vi "parseCommand.vi"(8 "error in (no error)":errorcluster, 10 "CMDString":string, 11 "CommandParser in":refnum<class "CommandParser.lvclass">) -> (0 "error out":errorcluster, 1 "parameter":variant, 2 "MonoCommand":T1, 3 "CommandParser out":refnum<class "CommandParser.lvclass">)   [LabVIEW 2016, in "CommandParser.lvclass"]
uses:
  CommandParser.lvclass
  Typedefs/MonoCommand.ctl
  Typedefs/wavelength.ctl
  Typedefs/slitPosition.ctl
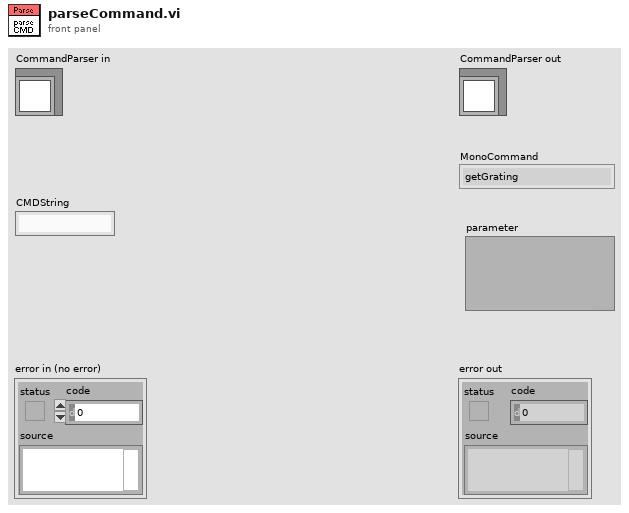
[diagram p1: front panel]
types:
  T1 = typedef "MonoCommand.ctl" = enum16{"getGrating", "getFrontEntranceSlitPosition", "getFrontExitSlitPosition", "getWavelength", "setWavelength", "setGrating", "setFrontEntranceSlitPosition", "setFrontExitSlitPosition", "calibrateWavelength", "Unknown"}
  T2 = typedef "wavelength.ctl" = dbl
  T3 = typedef "slitPosition.ctl" = dbl
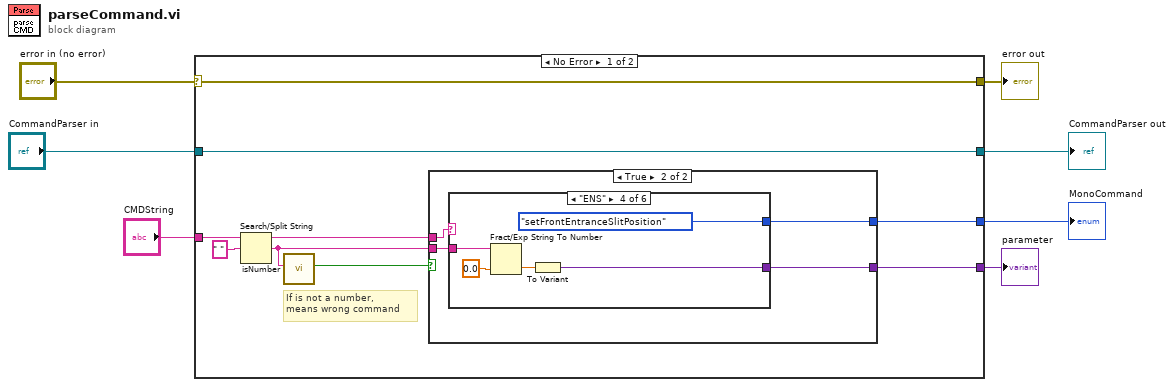
[diagram p0: block diagram]
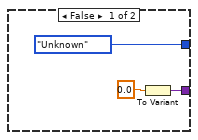
[diagram p2: hidden frame]
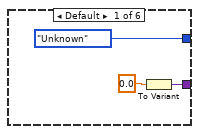
[diagram p3: hidden frame]
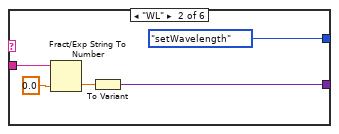
[diagram p4: hidden frame]
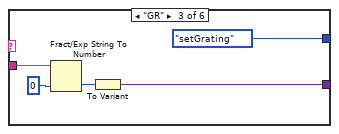
[diagram p5: hidden frame]
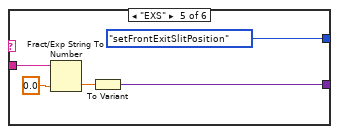
[diagram p6: hidden frame]
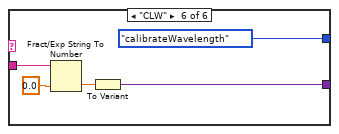
[diagram p7: hidden frame]
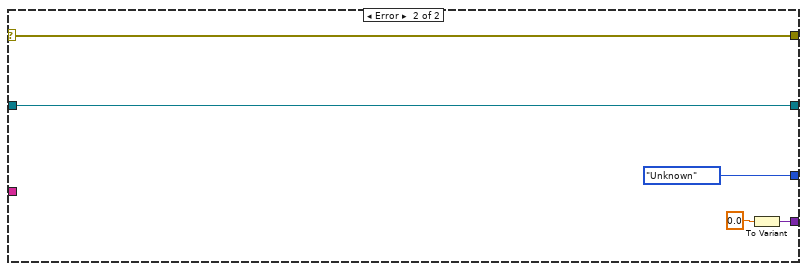
[diagram p8: hidden frame]
diagram:
  n1 = case shown="No Error" "error in (no error)" {
    selector: "error in (no error)" -> [w15 w56]
    tunnel: [w15 w56] -> w6
    tunnel: [w16 w55] -> w4
    tunnel: "CommandParser in" -> [w16 w55]
    tunnel: "CMDString" -> [w13 _]
    tunnel: [w14 MonoCommand."Unknown" ("MonoCommand")] -> w2
    tunnel: [w10 w52] -> w1
    frame No Error {
      # "If is not a number, \nmeans wrong command"
      n2 = Search/Split String(string=w13, search string/char (-)=" ") -> (substring before match=w11:string, match + rest of string=w8:string)  [unwired: 1 in, 1 out]
      n3 = call "isNumber.vi"("string"=w8) -> ("isNumber?"=w9:bool)  [unwired: 8 in, 2 out]
      n4 = case shown="True" w9 {
        tunnel: [MonoCommand."Unknown" ("MonoCommand") w23] -> w14
        tunnel: w11 -> [_ w22]
        tunnel: [w18 w21] -> w10
        tunnel: w8 -> [_ w20]
        frame False {
          n5 = To Variant(anything=T2 0.0 ("wavelength")) -> (Variant=w18:variant)
        }
        frame True {
          n6 = case shown="\"ENS\"" w22 {
            tunnel: [MonoCommand."Unknown" ("MonoCommand") MonoCommand."setWavelength" ("MonoCommand") MonoCommand."setGrating" ("MonoCommand") MonoCommand."setFrontEntranceSlitPosition" ("MonoCommand") MonoCommand."setFrontExitSlitPosition" ("MonoCommand") MonoCommand."calibrateWavelength" ("MonoCommand")] -> w23
            tunnel: w20 -> [_ w31 w36 w40 w43 w51]
            tunnel: [w24 w29 w32 w41 w44 w48] -> w21
            frame Default {
              n7 = To Variant(anything=T2 0.0 ("wavelength")) -> (Variant=w24:variant)
            }
            frame "WL" {
              n8 = Fract/Exp String To Number(string=w31, default (0 dbl)=T2 0.0 ("wavelength")) -> (number=w27:dbl)  [unwired: 2 in, 1 out]
              n9 = To Variant(anything=w27) -> (Variant=w29:variant)
            }
            frame "GR" {
              n10 = Fract/Exp String To Number(string=w36, default (0 dbl)=u16 0) -> (number=w33:u16)  [unwired: 2 in, 1 out]
              n11 = To Variant(anything=w33) -> (Variant=w32:variant)
            }
            frame "ENS" {
              n12 = Fract/Exp String To Number(string=w40, default (0 dbl)=T3 0.0 ("position")) -> (number=w39:dbl)  [unwired: 2 in, 1 out]
              n13 = To Variant(anything=w39) -> (Variant=w41:variant)
            }
            frame "EXS" {
              n14 = Fract/Exp String To Number(string=w43, default (0 dbl)=T3 0.0 ("position")) -> (number=w45:dbl)  [unwired: 2 in, 1 out]
              n15 = To Variant(anything=w45) -> (Variant=w44:variant)
            }
            frame "CLW" {
              n16 = Fract/Exp String To Number(string=w51, default (0 dbl)=T2 0.0 ("wavelength")) -> (number=w47:dbl)  [unwired: 2 in, 1 out]
              n17 = To Variant(anything=w47) -> (Variant=w48:variant)
            }
          }
        }
      }
    }
    frame Error {
      n18 = To Variant(anything=T2 0.0 ("wavelength")) -> (Variant=w52:variant)
    }
  }
  "error out" <- w6
  "CommandParser out" <- w4
  "MonoCommand" <- w2
  "parameter" <- w1
